vi "Toggle Button.vi"(11 "Boolean in":bool) -> (3 "Boolean out":bool)   [LabVIEW 2019]
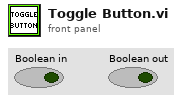
[diagram p1: front panel]
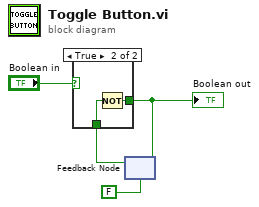
[diagram p0: block diagram]
diagram:
  n1 = feedback #1(FALSE) -> (w1:bool)
  n2 = case shown="True" "Boolean in" {
    tunnel: w1 -> [w5 w7]
    tunnel: [w5 w6] -> w4
    frame False {
    }
    frame True {
      n3 = Not(x=w7) -> (.not. x?=w6:bool)
    }
  }
  "Boolean out" <- w4
  n4 = feedback-in #1(w4) -> ()
